vi "OpenFile.vi"(8 "error in (no error)":errorcluster, 10 "File Path":path, 11 "ROFile in":refnum<class "WOFile.lvclass">) -> (0 "error out":errorcluster, 3 "WOFile out":refnum<class "WOFile.lvclass">)   [LabVIEW 2021, in "WOFile.lvclass"]
uses:
  WOFile.lvclass
  WOFile.lvclass/WOFile.ctl
  File/File.lvclass
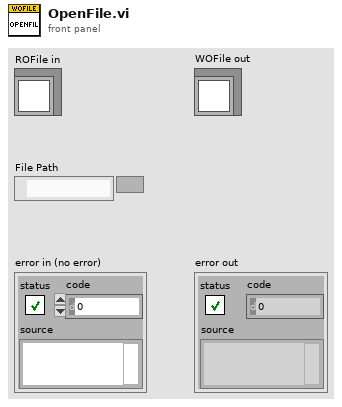
[diagram p1: front panel]
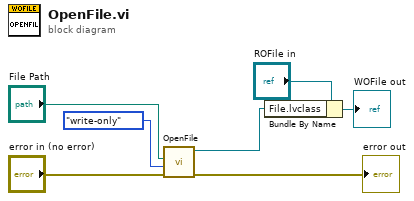
[diagram p0: block diagram]
diagram:
  n1 = call "OpenFile.vi"("error in (no error)"="error in (no error)", "access (0:read/write)"=enum16{"read/write", "read-only", "write-only"}."write-only", "File Path"="File Path") -> ("error out"=→"error out":errorcluster, "File out"=w1:refnum<class "File.lvclass">)  [unwired: 7 in]
  n2 = Bundle By Name(cluster="ROFile in", "File.lvclass"=w1) -> (→"WOFile out":refnum<class "WOFile.lvclass">)
